vi "uBroker_get_LastValue.vi"(6 "timeout in ms (1000)":i32=1000, 8 "error in (no error)":errorcluster, 10 "topic":string, 11 "uBroker in":refnum<class "uTransport_uActor.lvclass">) -> (0 "error out":errorcluster, 1 "Last Published Event":refnum<class "uMsg.lvclass">)   [LabVIEW 2023, in "uFramework.lvlib" / "uBroker.lvclass"]
doc: "This is a dataflow blocking message that is used to read the last published event on the specified topic."
uses:
  uBroker.lvclass
  uTransport_uActor/uTransport_uActor.lvclass
  U:/Projects/uFramework/Src/uFramework/uTransport/uTransport.lvclass
  uMsg/uMsg.lvclass
  Bin/uData.lvlibp/uData.lvclass
  uTransport_Queue/uTransport_Queue.lvclass/uTransport_Queue.ctl
  uMsg/uMsg.lvclass/uMsg.ctl
  uMsg/uMsg Create.vi
  uMsg/uMsg Get Payload.vi
  uTransport/uTransport_SendMsg.vi
  uTransport_Queue/uTransport_Queue_Create.vi
  uMsg/uMsg Update Timestamp.vi
  uTransport_Queue/uTransport_Queue.lvclass
  <vilib>/Utility/error.llb/Error Cluster From Error Code.vi
  uTransport/uTransport.lvclass
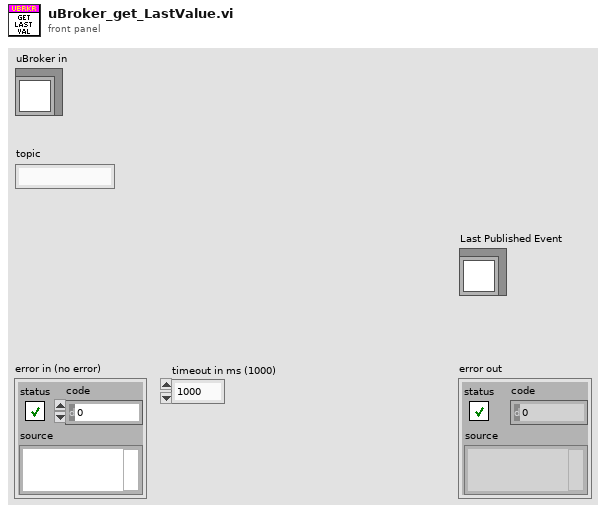
[diagram p1: front panel]
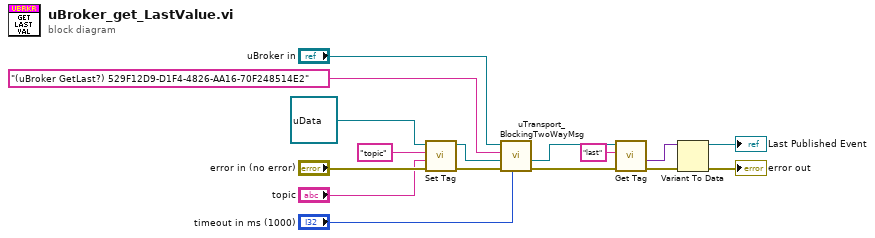
[diagram p0: block diagram]
diagram:
  n1 = call "Set Tag.vi"("error in (no error)"="error in (no error)", "Variant"="topic", "tag (case insensitive)"="topic", "uData in"=refnum<class "uData.lvclass"> refnum) -> ("error out"=w8:errorcluster, "uData out"=w7:refnum<class "uData.lvclass">)  [unwired: 5 in, 1 out]
  n2 = call "uTransport_BlockingTwoWayMsg.vi"("timeout in ms (5000)"="timeout in ms (1000)", "error in (no error)"=w8, "Data"=w7, "Command"="(uBroker GetLast?) 529F12D9-D1F4-4826-AA16-70F248514E2", "uTransport in"="uBroker in") -> ("error out"=w13:errorcluster, "Reply"=w2:refnum<class "uData.lvclass">)  [unwired: 5 in]
  n3 = call "Get Tag.vi"("error in (no error)"=w13, "tag (case insensitive)"="last", "uData in"=w2) -> ("error out"=w11:errorcluster, "value"=w1:variant)  [unwired: 5 in, 2 out]
  n4 = Variant To Data(error in=w11, Variant=w1) -> (data=→"Last Published Event":refnum<class "uMsg.lvclass">, error out=→"error out":errorcluster)  [unwired: 1 in]
